vi "Configure Source Range.vi"(8 "error in (no error)":errorcluster, 9 "Source Range (1.0)":dbl=1.0, 10 "Function (0: Volts)":u16(ring) items=["Volts", "Current"], 11 "VISA resource name":refnum<visa-resource-name>) -> (0 "error out":errorcluster, 3 "VISA resource name out":refnum<visa-resource-name>)   [LabVIEW 2021, in "Keithley 2450.lvlib"]
doc: "Configures the source range on the instrument."
uses:
  <instrlib>/Keithley 2450/Keithley 2450.lvlib
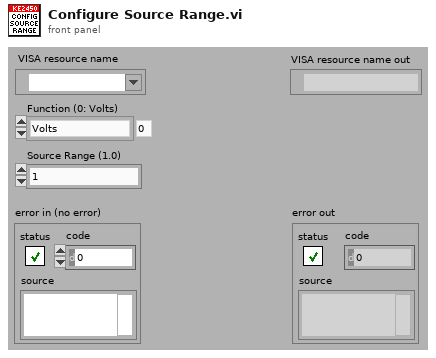
[diagram p1: front panel]
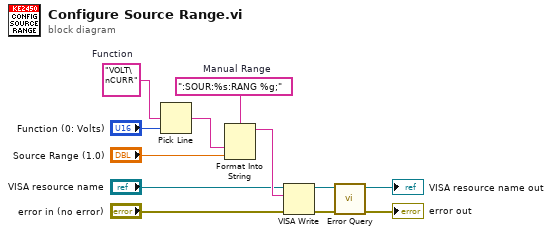
[diagram p0: block diagram]
diagram:
  w5 = "VOLT\nCURR"  # Function
  w7 = ":SOUR:%s:RANG %g;"  # Manual Range
  n1 = Pick Line(multi-line string=w5, line index="Function (0: Volts)") -> (output string=w3:string)  [unwired: 1 out]
  n2 = Format Into String(format string=w7, w3, "Source Range (1.0)") -> (resulting string=w8:string)  [unwired: 2 in, 1 out]
  n3 = VISA Write(VISA resource name="VISA resource name", write buffer=w8, error in (no error)="error in (no error)") -> (VISA resource name out=w10:refnum<visa-resource-name>, error out=w9:errorcluster)  [unwired: 1 out]
  n4 = call <instrlib>:"Error Query.vi"("error in (no error)"=w9, "VISA resource name"=w10) -> ("error out"=→"error out":errorcluster, "VISA resource name out"=→"VISA resource name out":refnum<visa-resource-name>)  [unwired: 8 out]
